vi "Is Empty VCluster__ogtk.vi"(1 "Variant":variant) -> (0 "Empty VCluster?":bool)   [LabVIEW 2023, in "openg_variant.lvlib"]
uses:
  openg_variant.lvlib
panel:
  # "EXPERIMENTAL"
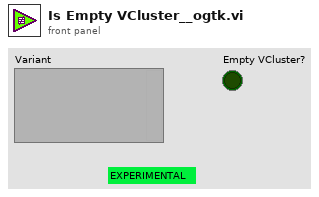
[diagram p1: front panel]
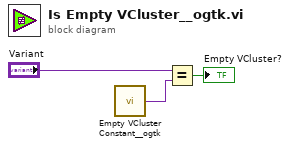
[diagram p0: block diagram]
diagram:
  n1 = call "Empty VCluster Constant__ogtk.vi"() -> ("Empty Cluster"=w2:variant)
  n2 = Equal?(x="Variant", y=w2) -> (x = y?=→"Empty VCluster?":bool)
